vi "MecaDrivePoseEst_Kalman_F_Callback.vi"(9 "U":T1, 10 "X":T1, 11 "ExtraPassedData":variant) -> (0 "Error":bool, 3 "Result":T1)   [LabVIEW 2019, in "Trajectory_Library.lvlib"]
doc: "Meca Drive Pose Estimator, Kalman Filter F function. \n\nThis function returns the U matrix.\n\nInput:\n - ExtraPassedData -- Variant contaiing extra data for the callback For this function the extra data should be empty..\n - X Matrix -- X matrix\n - U Matrix -- U matrix\n\nOutput:\n - Result -- Matrix resulting from calculation\n - Error -- If TRUE an error occured"
uses:
  <vilib>/Analysis/Matrix/Datatypes/RealMatrix.ctl
  Trajectory_Library.lvlib
  <vilib>/Analysis/Matrix/NI_Matrix.lvlib
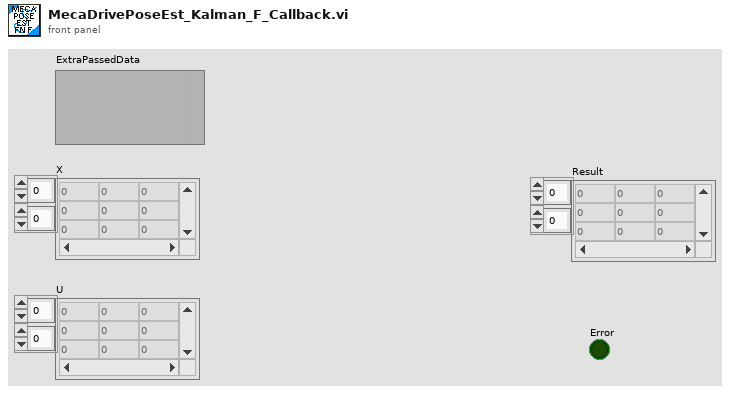
[diagram p1: front panel]
types:
  T1 = typedef "NI_Matrix.lvlib/RealMatrix.ctl" = dbl[][]
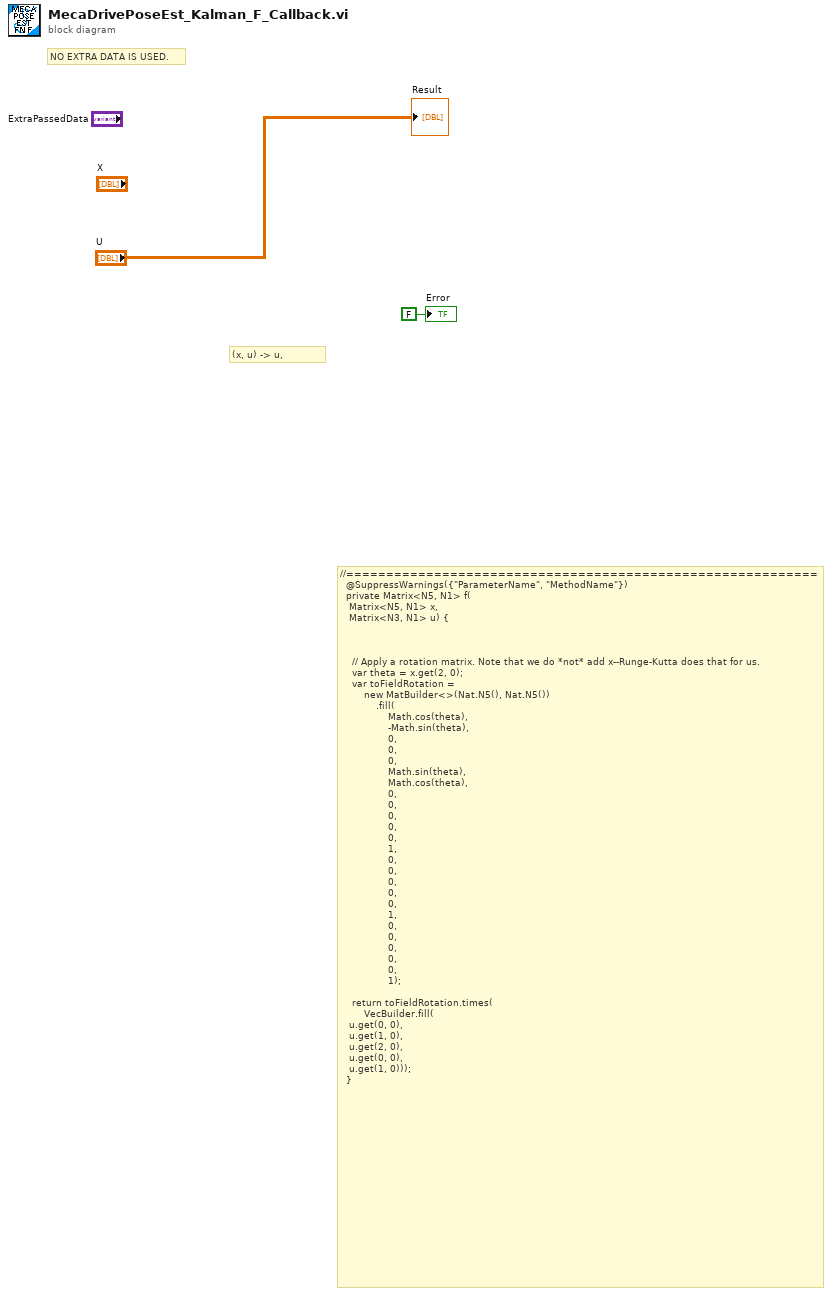
[diagram p0: block diagram]
diagram:
  # "(x, u) -> u,"
  # "NO EXTRA DATA IS USED."
  # "//===========================================================\n  @SuppressWarnings({\"ParameterName\", \"MethodName\"})\n  private Matrix<N5, N1> f(\n\t\t\tMatrix<N5, N1> x, \n\t\t\tMatrix<N3, N1> u) {\n\n\n\n    // Apply a rotation matrix. Note that we do *not* add x--Runge-Kutta does that for us.\n    var theta = x.get(2, 0);\n    var toFieldRotation =\n        new MatBuilder<>(Nat.N5(), Nat.N5())\n            .fill(\n                Math.cos(theta),\n                -Math.sin(theta),\n                0,\n                0,\n                0,\n                Math.sin(theta),\n                Math.cos(theta),\n                0,\n                0,\n                0,\n                0,\n                0,\n                1,\n                0,\n                0,\n                0,\n                0,\n                0,\n                1,\n                0,\n                0,\n                0,\n                0,\n                0,\n                1);\n\n    return toFieldRotation.times(\n        VecBuilder.fill(  \n\t\t\tu.get(0, 0), \n\t\t\tu.get(1, 0), \n\t\t\tu.get(2, 0), \n\t\t\tu.get(0, 0), \n\t\t\tu.get(1, 0)));\n  }"
  "Result" <- "U"
  "Error" <- FALSE ("Error")
